vi "testCam.vi"() -> ()   [LabVIEW 2019]
uses:
  <vilib>/userDefined/High Color/IMAQdx.ctl
  <vilib>/Platform/TimedLoop/XDataNode/timing_clust.ctl
  <vilib>/Platform/TimedLoop/XDataNode/nitl_modes.ctl
  <vilib>/Platform/TimedLoop/XDataNode/wakeup.ctl
  <vilib>/platform/TimedLoop/XDataNode/XDataNode.xnode
  <vilib>/vision/driver/NI_Vision_Acquisition_Software.lvlib
  <vilib>/Platform/TimedLoop/XDataNode/XDNodeRunTimeDep.lvlib
panel:
  out "diff number frame":u32(graph)
  in  "Boolean":bool
  out "picture":T1(plugin-control)
  out "dt":u32(graph)
  out "error out":errorcluster
  in  "stop":bool
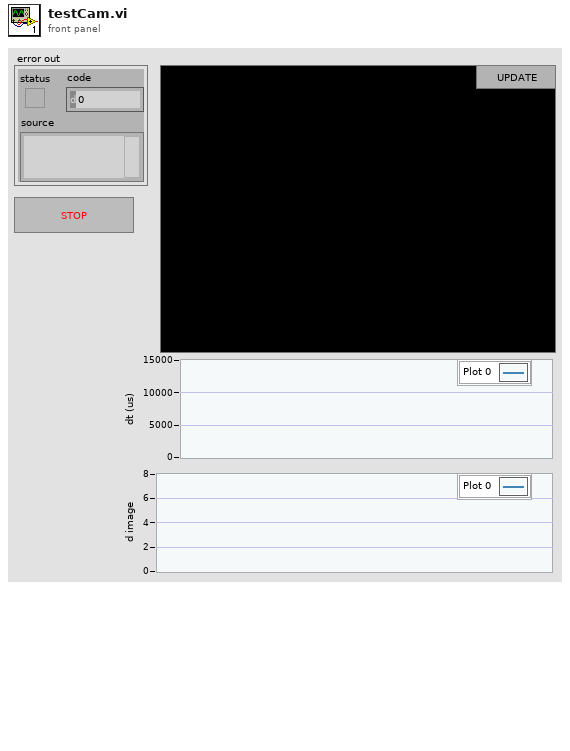
[diagram p1: front panel]
types:
  T1 = typedef "IMAQ Image.ctl" = refnum<image>
  T2 = typedef "IMAQdx.ctl" = refnum<k21>
  T3 = typedef "XDNodeRunTimeDep.lvlib/timing_clust.ctl" = cluster{"Expected End [f-1]":u64, "Actual End [f-1]":u64, "Finished Late? [f-1]":bool, "Expected End [i-1]":u64, "Actual End [i-1]":u64, "Finished Late? [i-1]":bool, "Expected Start [i]":u64, "Actual Start [i]":u64, "Expected Start [f]":u64, "Actual Start [f]":u64, "Source Name":string, "Structure Name":string, "Period":i64, "Deadline":i64, "Offset":i64, "Start":i64, "Priority":i32, "Timeout":i32, "Mode":T4, "Wakeup Reason":T5, "Error":errorcluster, "Source Type":string, "Secondary Source Type":string, "Global End Time":u64, "Global Start Time":u64, "Frame Duration":u64, "Iteration Duration":u64, "Assigned CPU":i32, "I/O Scan Engine Mode":u32}
  T4 = typedef "XDNodeRunTimeDep.lvlib/nitl_modes.ctl" = enum32{"No Change", "Process missed periods, maintain original phase", "Discard missed periods, maintain original phase", "Process missed periods, ignore original phase", "Discard missed periods, ignore original phase"}
  T5 = typedef "XDNodeRunTimeDep.lvlib/wakeup.ctl" = enum32{"Normal", "Aborted", "Asynchronous wakeup", "Timing source error", "Timed loop error", "Timeout"}
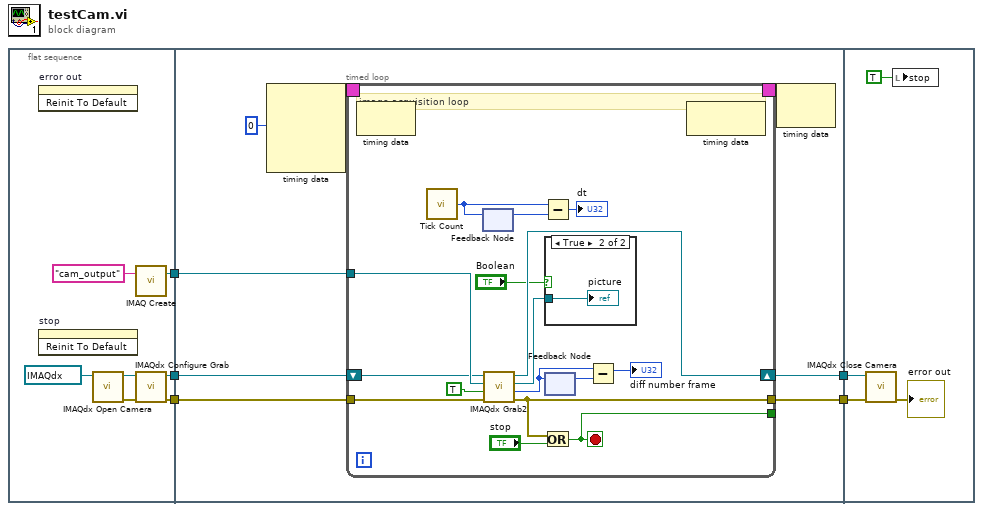
[diagram p0: block diagram]
diagram:
  n1 = flat-sequence {
    tunnel: [w8] -> w4
    tunnel: [w6] -> w3
    tunnel: [w7] -> w2
    tunnel: [w17] -> w5
    tunnel: w4 -> [w20]
    tunnel: w3 -> [w19]
    tunnel: w2 -> [w18]
    tunnel: [w16] -> w1
    tunnel: w5 -> [w45]
    tunnel: w1 -> [w46]
    frame #0 {
      n2 = invoke on="error out" class="Clust (strict)" method="Reinit To Default"() -> ()  [unwired: 3 in, 3 out]
      n3 = invoke on="stop" class="Bool (strict)" method="Reinit To Default"() -> ()  [unwired: 3 in, 3 out]
      n4 = call <vilib>:"IMAQdx Open Camera.vi"("Session In"=T2 "cam2") -> ("error out"=w12:errorcluster, "Session Out"=w11:T2)  [unwired: 9 in]
      n5 = call "IMAQ Create"("Image Name"="cam_output") -> ("New Image"=w8:T1)  [unwired: 4 in, 1 out]
      n6 = call <vilib>:"IMAQdx Configure Grab.vi"("error in"=w12, "Session In"=w11) -> ("error out"=w7:errorcluster, "Session Out"=w6:T2)  [unwired: 8 in]
    }
    frame #1 {
      n7 = node-c288(i64 0 ("Period")) -> (w15:T3)  [unwired: 3 in]
      n8 = timed-loop {
        tunnel: w20 -> [w34]
        shift-right: [w36] -> w16
        shift-left: w19 -> [w33]
        tunnel: w18 -> [w32]
        tunnel: [w31] -> _
        tunnel: [w30] -> w17
        timing: w15 -> [_]
        timing-out: [_] -> w14
        stop <- w31 stop-if-true
        # "image acquisition loop"
        n9 = node-c288() -> ()  [unwired: 1 in, 1 out]
        n10 = call "Tick Count"() -> ("Tick Count(uSec)"=w28:u32)
        n11 = feedback-in #1(w28) -> ()
        n12 = feedback #1() -> (w35:u32)  [unwired: 1 in]
        n13 = call <vilib>:"IMAQdx Grab2.vi"("error in"=w32, "Wait for Next Buffer? (Yes)"=TRUE, "Image In"=w34, "Session In"=w33) -> ("error out"=w30:errorcluster, "Buffer Number Out"=w23:u32, "Image Out"=w29:T1, "Session Out"=w36:T2)  [unwired: 4 in]
        n14 = Subtract(x=w28, y=w35) -> (x-y=→"dt":u32)
        n15 = Or(x=w30, y="stop") -> (x .or. y?=w31:bool)
        n16 = case shown="True" "Boolean" {
          tunnel: w29 -> [_ w39]
          frame False {
          }
          frame True {
            "picture" <- w39
          }
        }
        n17 = feedback #2() -> (w24:u32)  [unwired: 1 in]
        n18 = feedback-in #2(w23) -> ()
        n19 = Subtract(x=w23, y=w24) -> (x-y=→"diff number frame":u32)
        n20 = node-c288() -> ()  [unwired: 1 in, 1 out]
      }
      n21 = node-c288(w14) -> ()  [unwired: 1 out]
    }
    frame #2 {
      n22 = call <vilib>:"IMAQdx Close Camera.vi"("error in"=w45, "Session In"=w46) -> ("error out"=→"error out":errorcluster)  [unwired: 9 in]
      n23 = local write "stop"(TRUE ("stop")) -> ()
    }
  }
